vi "Initialize.vi"(8 "error in":errorcluster, 10 "parameters":variant, 11 "node in":refnum<class "ThreePhasePLL editor node.lvclass">) -> (0 "error out":errorcluster, 2 "summary":T2[](array[typedef]), 3 "data value reference":T1)   [LabVIEW 2017, in "ThreePhasePLL editor node.lvclass"]
doc: "Initializes the data of a node to its default state.\nThe object is not created inside of this VI, because it is created from a File depending on user selection."
uses:
  ThreePhasePLL editor node.lvclass
  C:/Program Files (x86)/National Instruments/LabVIEW 2017/vi.lib/NI/Configuration Framework/Node/NISE_CEF_Node.lvclass
  <vilib>/NI/Configuration Framework/Node/Summary.ctl
  <vilib>/NI/Configuration Framework/Node/NodeRef.ctl
  <vilib>/NI/Configuration Framework/Node/NISE_CEF_Node.lvclass
  <vilib>/NI/PowerElectronicsControl/ThreePhasePLL/Interface/Configuration.ctl
  <vilib>/rvi/Analysis/control/PID/Typedef/niFpgaPID_PIGains.ctl
  <vilib>/rvi/Analysis/control/PID/Typedef/niFpgaPID_OutputRange.ctl
  module/configuration/ThreePhasePLL configuration.lvclass
  C:/Program Files (x86)/National Instruments/LabVIEW 2017/vi.lib/NI/Configuration Framework/serializable configuration/NISE_CEF_serializable configuration.lvclass
  module/configuration/ThreePhasePLL configuration.lvclass/ThreePhasePLL configuration.ctl
  <vilib>/NI/DCAF/Tag Editor Core/control module/editor node/control module editor.lvclass
  <vilib>/NI/Configuration Framework/serializable configuration/NISE_CEF_serializable configuration.lvclass
  <vilib>/NI/PowerElectronicsControl/ThreePhasePLL/Interface/ThreePhasePLLInterface.lvlib
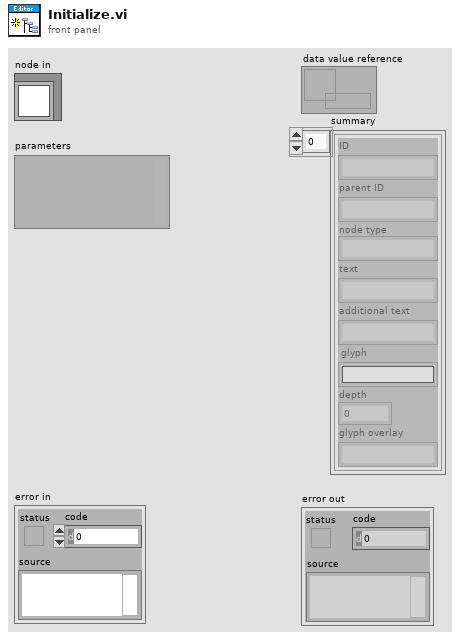
[diagram p1: front panel]
types:
  T1 = typedef "NISE_CEF_Node.lvclass/NodeRef.ctl" = refnum<data-value>
  T2 = typedef "NISE_CEF_Node.lvclass/Summary.ctl" = cluster{"ID":string, "parent ID":string, "node type":string, "text":string, "additional text":string, "glyph":string, "depth":i32, "glyph overlay":string}
  T3 = typedef "ThreePhasePLLInterface.lvlib/Configuration.ctl" = cluster{"PLLgains":T4, "PLLrange":T5, "dT":sgl, "expectedFreq":sgl, "lockDuration":sgl, "freqBoundaries":sgl}
  T4 = typedef "niFpgaPID_PIGains.ctl" = cluster{"proportional gain":sgl, "integral gain":sgl}
  T5 = typedef "niFpgaPID_OutputRange.ctl" = cluster{"output high (Inf)":sgl, "output low (-Inf)":sgl}
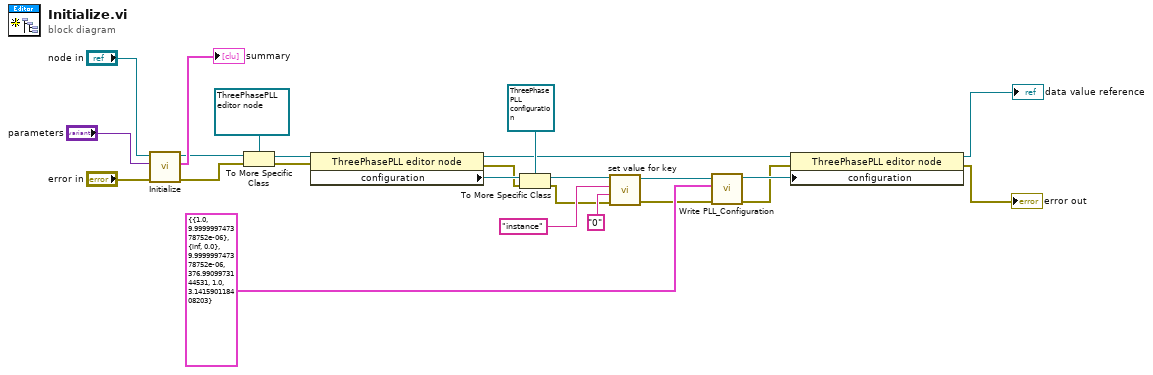
[diagram p0: block diagram]
diagram:
  n1 = call-parent "Initialize.vi"("error in"="error in", "parameters"="parameters", "node in"="node in") -> ("error out"=w19:errorcluster, "summary"=→"summary":T2[], "data value reference"=w20:T1)  [unwired: 6 in]
  n2 = To More Specific Class(target class=refnum<data-value> refnum ("data value reference"), reference=w20, error in=w19) -> (specific class reference=w17:refnum<data-value>, error out=w16:errorcluster)
  n3 = property class="ThreePhasePLL editor node"(reference=w17, error in=w16) -> (reference out=w11:refnum<data-value>, error out=w13:errorcluster, "configuration"=w14:refnum<class "NISE_CEF_serializable configuration.lvclass">)
  n4 = To More Specific Class(target class=refnum<class "ThreePhasePLL configuration.lvclass"> refnum ("ThreePhasePLL configuration"), reference=w14, error in=w13) -> (specific class reference=w4:refnum<class "ThreePhasePLL configuration.lvclass">, error out=w1:errorcluster)
  n5 = call-dynamic "set value for key.vi"("error in"=w1, "value"="0", "key"="instance", "fixed channel configuration in"=w4) -> ("error out"=w2:errorcluster, "fixed channel configuration out"=w3:refnum<class "ThreePhasePLL configuration.lvclass">)  [unwired: 6 in]
  n6 = call "Write PLL_Configuration.vi"("error in (no error)"=w2, "Configuration"=T3 {"PLLgains"={"proportional gain"=1.0, "integral gain"=1e-05}, "PLLrange"={"output high (Inf)"=inf, "output low (-Inf)"=0.0}, "dT"=1e-05, "expectedFreq"=376.991, "lockDuration"=1.0, "freqBoundaries"=3.14159}, "ThreePhasePLL configuration in"=w3) -> ("error out"=w9:errorcluster, "ThreePhasePLL configuration out"=w10:refnum<class "ThreePhasePLL configuration.lvclass">)  [unwired: 7 in]
  n7 = property class="ThreePhasePLL editor node"(reference=w11, error in=w9, "configuration"=w10) -> (reference out=→"data value reference":refnum<data-value>, error out=→"error out":errorcluster)
